vi "XLM_SetupXMLValue.vi"(0 "ValueUnit":string(combo), 1 "Name":string, 2 "Max":string, 3 "Value":string, 4 "Min":string, 5 "Uint":string, 6 "Status":string) -> (20 "生成的XML 2":string)   [LabVIEW 2018]
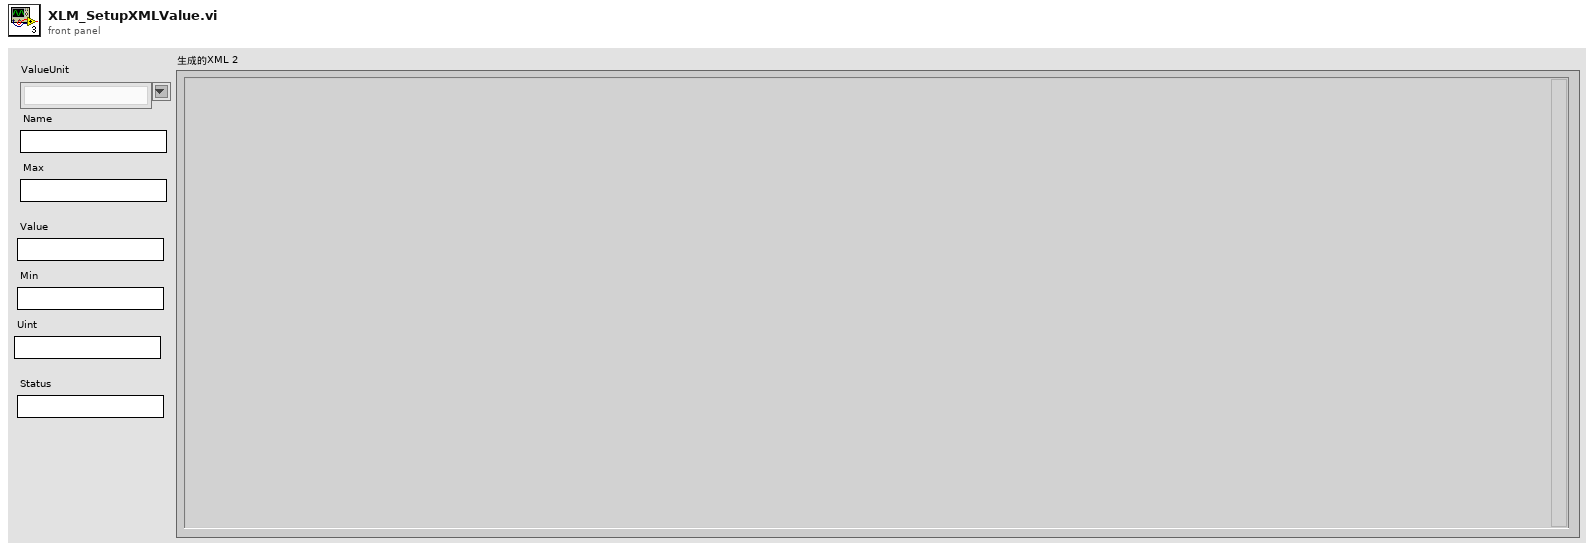
[diagram p1: front panel]
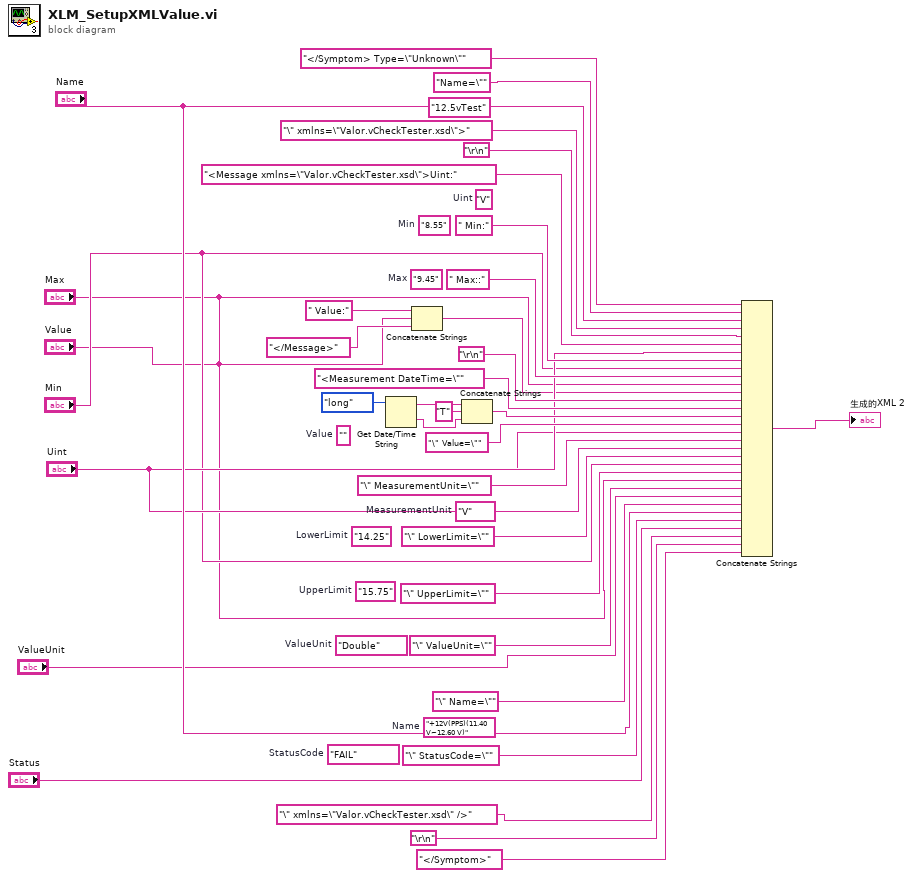
[diagram p0: block diagram]
diagram:
  (unwired) "FAIL"  # StatusCode
  (unwired) "+12V(PPS)(11.40 V~12.60 V)"  # Name
  (unwired) "Double"  # ValueUnit
  (unwired) "15.75"  # UpperLimit
  (unwired) "14.25"  # LowerLimit
  (unwired) "V"  # MeasurementUnit
  (unwired) ""  # Value
  (unwired) "9.45"  # Max
  (unwired) "8.55"  # Min
  (unwired) "V"  # Uint
  (unwired) "12.5vTest"
  n1 = Get Date/Time String(date format (0)=enum16{"short", "long", "abbreviated"}."long" ("日期格式(0)")) -> (date string=w24:string, time string=w23:string)  [unwired: 2 in]
  n2 = Concatenate Strings(" Value:" ("字符串"), "Value", "</Message>" ("字符串")) -> (w3:string)
  n3 = Concatenate Strings(w24, "T" ("字符串"), w23) -> (w22:string)
  n4 = Concatenate Strings("</Symptom> Type=\"Unknown\"", "Name=\"", "Name", "\" xmlns=\"Valor.vCheckTester.xsd\">" ("字符串"), "\r\n", "<Message xmlns=\"Valor.vCheckTester.xsd\">Uint:" ("字符串"), "Uint", " Min:" ("字符串"), "Min", " Max::" ("字符串"), "Max", w3, "\r\n", "<Measurement DateTime=\"" ("字符串"), w22, "\" Value=\"" ("字符串"), "Value", "\" MeasurementUnit=\"" ("字符串"), "Uint", "\" LowerLimit=\"" ("字符串"), "Min", "\" UpperLimit=\"" ("字符串"), "Max", "\" ValueUnit=\"" ("字符串"), "ValueUnit", "\" Name=\"" ("字符串"), "Name", "\" StatusCode=\"" ("字符串"), "Status", "\" xmlns=\"Valor.vCheckTester.xsd\" />" ("字符串"), "\r\n", "</Symptom>") -> (→"生成的XML 2":string)
